vi "RT 16 bit DAC.vi"() -> ()   [LabVIEW 2018]
doc: "The myRIO Custom FPGA Project template acquires button data from the onboard button and displays the button value on a Boolean indicator. The SYS.RDY indicator shows the FPGA status."
uses:
  <vilib>/Platform/TimedLoop/XDataNode/timing_clust.ctl
  <vilib>/Platform/TimedLoop/XDataNode/nitl_modes.ctl
  <vilib>/Platform/TimedLoop/XDataNode/wakeup.ctl
  <vilib>/FPGAPlugInAG/myRIO-1900/niLvFpga_Open_myRIO-1900.vi
  <vilib>/rvi/interface/common/dynamic/niFpgaDynamicAddResources.vi
  <vilib>/Utility/error.llb/Error Cluster From Error Code.vi
  <vilib>/rvi/errors/niLvFpgaAdjustHostInterfaceError.vi
  <vilib>/FPGAPlugInAG/Dynamic/niLvFpga_Close_Dynamic.vi
  <vilib>/rvi/interface/nirviOpenFPGA/nirviOpenFPGA.xnode
  FPGA Bitfiles/ASPE2019StudentC_FPGATarget_FPGASPI_qic8khcfECQ.lvbitx
  FPGA_SPI.vi
  <vilib>/Platform/TimedLoop/XDataNode/XDataNode.xnode
  <vilib>/rvi/interface/nirviReadWriteControl/nirviReadWriteControl.xnode
  <vilib>/rvi/interface/nirviCloseFPGA/nirviCloseFPGA.xnode
  <vilib>/rvi/interface/Simulation/niFpgaSimulationCallBeginRW.vi
  <vilib>/Platform/TimedLoop/XDataNode/XDNodeRunTimeDep.lvlib
  NiFpgaLv.dll
panel:
  in  "milliseconds to wait":u32=10
  in  "Vout":dbl
  in  "DC OUT":bool
  in  "SPPC":u32=500
  out "Sample Rate(K/s)":dbl=0.5328524590163934 format="%#_8g"
  out "Freq (kHz)":dbl=0.001065704918032787 format="%.7g"
  in  "Amplitude":dbl=10.0 format="%0.3p"
  in  "Stop":bool
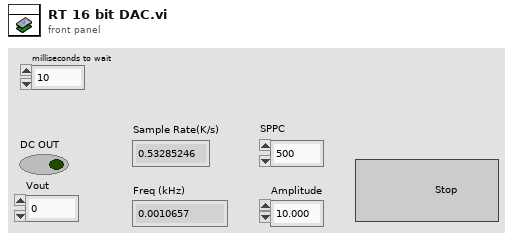
[diagram p1: front panel]
types:
  T1 = typedef "XDNodeRunTimeDep.lvlib/timing_clust.ctl" = cluster{"Expected End [f-1]":u64, "Actual End [f-1]":u64, "Finished Late? [f-1]":bool, "Expected End [i-1]":u64, "Actual End [i-1]":u64, "Finished Late? [i-1]":bool, "Expected Start [i]":u64, "Actual Start [i]":u64, "Expected Start [f]":u64, "Actual Start [f]":u64, "Source Name":string, "Structure Name":string, "Period":i64, "Deadline":i64, "Offset":i64, "Start":i64, "Priority":i32, "Timeout":i32, "Mode":T2, "Wakeup Reason":T3, "Error":errorcluster, "Source Type":string, "Secondary Source Type":string, "Global End Time":u64, "Global Start Time":u64, "Frame Duration":u64, "Iteration Duration":u64, "Assigned CPU":i32, "I/O Scan Engine Mode":u32}
  T2 = typedef "XDNodeRunTimeDep.lvlib/nitl_modes.ctl" = enum32{"No Change", "Process missed periods, maintain original phase", "Discard missed periods, maintain original phase", "Process missed periods, ignore original phase", "Discard missed periods, ignore original phase"}
  T3 = typedef "XDNodeRunTimeDep.lvlib/wakeup.ctl" = enum32{"Normal", "Aborted", "Asynchronous wakeup", "Timing source error", "Timed loop error", "Timeout"}
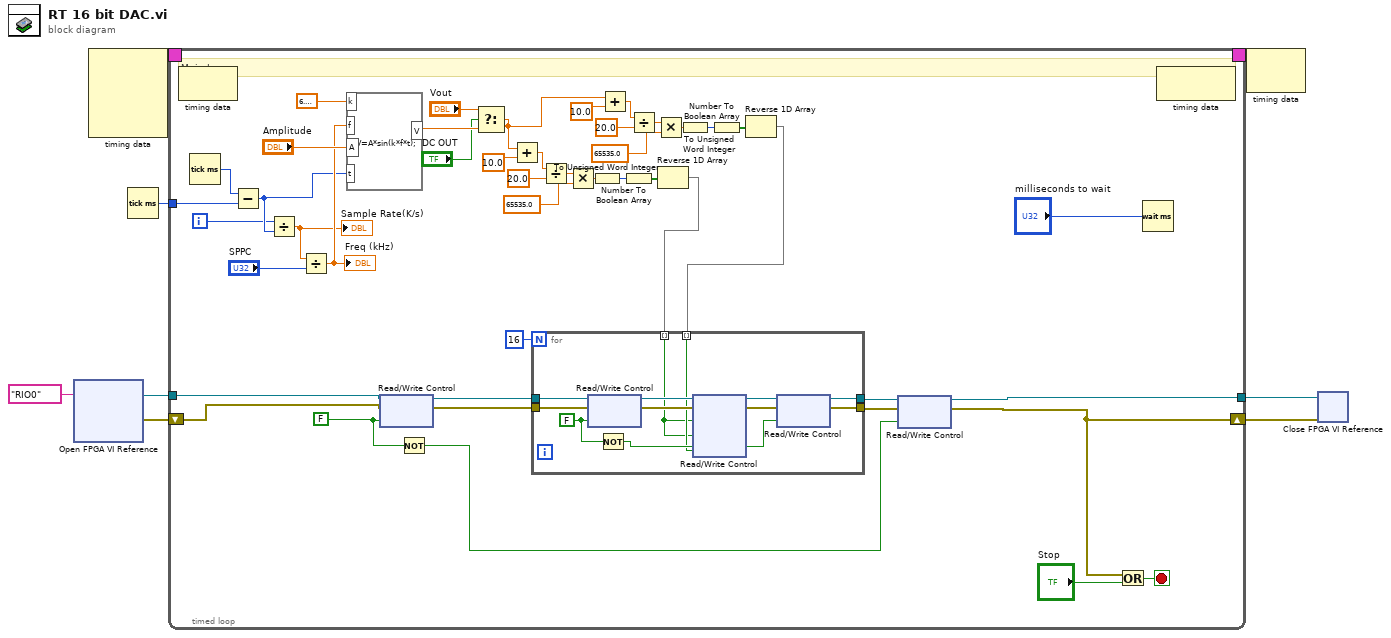
[diagram p0: block diagram]
diagram:
  n1 = xnode "Open FPGA VI Reference"("resource name"=tag "RIO0") -> ("FPGA VI Reference Out"=w6:refnum<k20>, "error out"=w5:errorcluster)  [unwired: 1 in]
  n2 = node-c288() -> (w2:T1)  [unwired: 4 in]
  n3 = Tick Count (ms)() -> (millisecond timer value=w3:u32)
  n4 = timed-loop {
    shift-right: [w30] -> w8
    shift-left: w5 -> [w19]
    tunnel: [w31] -> w7
    tunnel: w3 -> [w40]
    tunnel: w6 -> [w20]
    timing: w2 -> [_]
    timing-out: [_] -> w1
    i -> [w32]
    stop <- w52 stop-if-true
    w22 = FALSE ("CS")
    # "Main Loop"
    n5 = node-c288() -> ()  [unwired: 1 in, 1 out]
    n6 = Tick Count (ms)() -> (millisecond timer value=w34:u32)
    n7 = Subtract(x=w34, y=w40) -> (x-y=w48:u32)
    n8 = Divide(x=w32, y=w48) -> (x/y=w33:dbl)
    "Sample Rate(K/s)" <- w33
    n9 = Divide(x=w33, y="SPPC") -> (x/y=w49:dbl)
    "Freq (kHz)" <- w49
    n10 = formula code="V=A*sin(k*f*t);"("t"=w48, "f"=w49, "A"="Amplitude", "k"=6.283185307179586 ("input variable")) -> ("V"=w38:dbl)
    n11 = xnode "Read/Write Control"("FPGA VI Reference In"=w20, "error in"=w19, "CS"=w22) -> ("FPGA VI Reference Out"=w25:refnum<k20>, "error out"=w26:errorcluster)
    n12 = Not(x=w22) -> (.not. x?=w21:bool)
    n13 = Select(t="Vout", s="DC OUT", f=w38) -> (s? t:f=w10:dbl)
    n14 = Add(x=w10, y=10.0) -> (x+y=w45:dbl)
    n15 = Divide(x=w45, y=20.0) -> (x/y=w41:dbl)
    n16 = Multiply(x=w41, y=65535.0) -> (x*y=w42:dbl)
    n17 = To Unsigned Word Integer(number=w42) -> (unsigned 16bit integer=w43:u16)
    n18 = Add(x=w10, y=10.0) -> (x+y=w16:dbl)
    n19 = Number To Boolean Array(number=w43) -> (Boolean array=w35:bool[])
    n20 = Divide(x=w16, y=20.0) -> (x/y=w12:dbl)
    n21 = Multiply(x=w12, y=65535.0) -> (x*y=w13:dbl)
    n22 = Reverse 1D Array(array=w35) -> (reversed array=w28:bool[])
    n23 = To Unsigned Word Integer(number=w13) -> (unsigned 16bit integer=w14:u16)
    n24 = Number To Boolean Array(number=w14) -> (Boolean array=w11:bool[])
    n25 = Reverse 1D Array(array=w11) -> (reversed array=w9:bool[])
    n26 = for {
      N: 16 -> [_]
      tunnel: w25 -> [w65]
      tunnel: w26 -> [w64]
      tunnel: w28 -> [w54] mode=indexing
      tunnel: [w58] -> w24
      tunnel: [w57] -> w23
      tunnel: w9 -> [w55] mode=indexing
      w63 = FALSE ("CLK")
      n27 = xnode "Read/Write Control"("FPGA VI Reference In"=w65, "error in"=w64, "CLK2"=w63) -> ("FPGA VI Reference Out"=w62:refnum<k20>, "error out"=w61:errorcluster)
      n28 = Not(x=w63) -> (.not. x?=w56:bool)
      n29 = xnode "Read/Write Control"("FPGA VI Reference In"=w62, "error in"=w61, "MOSI2"=w54, "MOSI3"=w54, "MOSI4"=w55) -> ("FPGA VI Reference Out"=w60:refnum<k20>, "error out"=w59:errorcluster)
      n30 = xnode "Read/Write Control"("FPGA VI Reference In"=w60, "error in"=w59, "CLK2"=w56) -> ("FPGA VI Reference Out"=w58:refnum<k20>, "error out"=w57:errorcluster)
    }
    n31 = xnode "Read/Write Control"("FPGA VI Reference In"=w24, "error in"=w23, "CS"=w21) -> ("FPGA VI Reference Out"=w31:refnum<k20>, "error out"=w30:errorcluster)
    n32 = Or(x=w30, y="Stop") -> (x .or. y?=w52:bool)
    n33 = Wait (ms)(milliseconds to wait="milliseconds to wait") -> ()  [unwired: 1 out]
    n34 = node-c288() -> ()  [unwired: 1 in, 1 out]
  }
  n35 = node-c288(w1) -> ()  [unwired: 1 out]
  n36 = xnode "Close FPGA VI Reference"("FPGA VI Reference In"=w7, "error in"=w8) -> ()  [unwired: 1 out]
